vi "2_WF_Anomaly_Detection(Threshold_Evaluation).vi"() -> ()   [LabVIEW 2020]
uses:
  Controls/Optimal_Threshold_Range'.ctl
  <vilib>/Ngene/DeepLTK/Toolkit/NN_Network/subVIs/NN_Predict/NN_Predict(In1D_Out1D).vi
  <vilib>/Ngene/DeepLTK/Toolkit/NN_Data/subVIs/Get_Data_Vals/NN_Data_Get_ValByRef(2D_SGL).vi
  <vilib>/Ngene/DeepLTK/Toolkit/Deep_Learning_Toolkit_by_Ngene.lvlib
  <vilib>/Analysis/NI_AALPro.lvlib
panel:
  in  "Validation (Abnormal Samples) dataset path":path=path "D:/working/Anomaly Detection/Validation/Abnormal"
  in  "Validation (Normal Samples) dataset path":path=path "D:/working/Anomaly Detection/Validation/Normal"
  out "Integrals of Normalized Anomaly Score Distributions":cluster{"Axis":dbl[], "Integral X":dbl[]}[](graph)
  out "Anomaly Score Distribution":T1(graph)=[{"X Values"=array[700 elements], "Histogram: h(x)"=[0, 0, 0, 0, 0, 0, 0, 0, 0, 0, 0, 0, 0, 0, 0, 0, 0, 0, 0, 0, 0, 0, 0, 0, 0, 0, 0, 0, 0, 0, 0, 0, 0, 0, 0, 0, 1, 2, 5, 5, 8, 9, 5, 13, 9, 12, 13, 17, 13, 20, 12, 18, 18, 17, 20, 14, 17, 15, 19, 8, 9, 11, 14, 16, 9, 10, 16, 7, 6, 10, 10, 6, 9, 4, 4, 8, 3, 1, 5, 3, 2, 3, 5, 5, 3, 2, 3, 2, 2, 1, 4, 3, 0, 2, 0, 1, 1, 2, 3, 0, 1, 0, 0, 0, 0, 0, 0, 0, 0, 1, 0, 1, 1, 0, 0, 0, 0, 0, 0, 0, 1, 0, 0, 0, 0, 0, 0, 0, 0, 0, 0, 0, 0, 0, 0, 0, 0, 0, 0, 0, 0, 0, 0, 0, 0, 0, 0, 0, 0, 0, 0, 0, 0, 0, 0, 0, 0, 0, 0, 0, 0, 0, 0, 0, 0, 0, 0, 0, 0, 0, 0, 0, 0, 0, 0, 0, 0, 0, 0, 0, 0, 0, 0, 0, 0, 0, 0, 0, 0, 0, 0, 0, 0, 0, 0, 0, 0, 0, 0, 0, 0, 0, 0, 0, 0, 0, 0, 0, 0, 0, 0, 0, 0, 0, 0, 0, 0, 0, 0, 0, 0, 0, 0, 0, 0, 0, 0, 0, 0, 0, 0, 0, 0, 0, 0, 0, 0, 0, 0, 0, 0, 0, 0, 0, 0, 0, 0, 0, 0, 0, 0, 0, 0, 0, 0, 0, 0, 0, 0, 0, 0, 0, 0, 0, 0, 0, 0, 0, 0, 0, 0, 0, 0, 0, 0, 0, 0, 0, 0, 0, 0, 0, 0, 0, 0, 0, 0, 0, 0, 0, 0, 0, 0, 0, 0, 0, 0, 0, 0, 0, 0, 0, 0, 0, 0, 0, 0, 0, 0, 0, 0, 0, 0, 0, 0, 0, 0, 0, 0, 0, 0, 0, 0, 0, 0, 0, 0, 0, 0, 0, 0, 0, 0, 0, 0, 0, 0, 0, 0, 0, 0, 0, 0, 0, 0, 0, 0, 0, 0, 0, 0, 0, 0, 0, 0, 0, 0, 0, 0, 0, 0, 0, 0, 0, 0, 0, 0, 0, 0, 0, 0, 0, 0, 0, 0, 0, 0, 0, 0, 0, 0, 0, 0, 0, 0, 0, 0, 0, 0, 0, 0, 0, 0, 0, 0, 0, 0, 0, 0, 0, 0, 0, 0, 0, 0, 0, 0, 0, 0, 0, 0, 0, 0, 0, 0, 0, 0, 0, 0, 0, 0, 0, 0, 0, 0, 0, 0, 0, 0, 0, 0, 0, 0, 0, 0, 0, 0, 0, 0, 0, 0, 0, 0, 0, 0, 0, 0, 0, 0, 0, 0, 0, 0, 0, 0, 0, 0, 0, 0, 0, 0, 0, 0, 0, 0, 0, 0, 0, 0, 0, 0, 0, 0, 0, 0, 0, 0, 0, 0, 0, 0, 0, 0, 0, 0, 0, 0, 0, 0, 0, 0, 0, 0, 0, 0, 0, 0, 0, 0, 0, 0, 0, 0, 0, 0, 0, 0, 0, 0, 0, 0, 0, 0, 0, 0, 0, 0, 0, 0, 0, 0, 0, 0, 0, 0, 0, 0, 0, 0, 0, 0, 0, 0, 0, 0, 0, 0, 0, 0, 0, 0, 0, 0, 0, 0, 0, 0, 0, 0, 0, 0, 0, 0, 0, 0, 0, 0, 0, 0, 0, 0, 0, 0, 0, 0, 0, 0, 0, 0, 0, 0, 0, 0, 0, 0, 0, 0, 0, 0, 0, 0, 0, 0, 0, 0, 0, 0, 0, 0, 0, 0, 0, 0, 0, 0, 0, 0, 0, 0, 0, 0, 0, 0, 0, 0, 0, 0, 0, 0, 0, 0, 0, 0, 0, 0, 0, 0, 0, 0, 0, 0, 0, 0, 0, 0, 0, 0, 0, 0, 0, 0, 0, 0, 0, 0, 0, 0, 0, 0, 0, 0, 0, 0, 0, 0, 0, 0, 0, 0, 0, 0, 0, 0, 0, 0, 0, 0, 0, 0, 0, 0, 0, 0, 0, 0, 0, 0, 0, 0, 0, 0, 0, 0, 0, 0, 0, 0, 0, 0, 0, 0, 0, 0, 0, 0, 0, 0, 0, 0, 0, 0, 0, 0, 0, 0, 0, 0, 0, 0, 0]}, {"X Values"=array[700 elements], "Histogram: h(x)"=[0, 0, 0, 0, 0, 0, 0, 0, 0, 0, 0, 0, 0, 0, 0, 0, 0, 0, 0, 0, 0, 0, 0, 0, 0, 0, 0, 0, 0, 0, 0, 0, 0, 0, 0, 0, 0, 0, 0, 0, 0, 0, 0, 0, 0, 0, 0, 0, 0, 0, 0, 0, 0, 0, 0, 0, 0, 0, 0, 0, 0, 0, 0, 0, 0, 0, 0, 0, 0, 0, 0, 0, 0, 0, 0, 0, 0, 0, 0, 0, 0, 0, 0, 0, 0, 0, 0, 0, 0, 0, 0, 0, 0, 0, 0, 0, 0, 0, 0, 0, 0, 0, 0, 0, 0, 0, 0, 0, 0, 0, 0, 0, 0, 0, 0, 0, 0, 0, 0, 0, 0, 0, 0, 0, 0, 0, 0, 0, 0, 0, 0, 0, 0, 0, 0, 0, 0, 0, 0, 0, 0, 0, 0, 0, 0, 0, 0, 0, 0, 0, 0, 0, 0, 0, 0, 0, 0, 0, 0, 0, 0, 0, 0, 0, 0, 0, 0, 0, 0, 0, 0, 0, 1, 1, 0, 0, 0, 1, 0, 0, 1, 2, 2, 0, 0, 2, 1, 1, 2, 0, 0, 1, 2, 1, 2, 2, 1, 0, 1, 1, 2, 3, 0, 1, 2, 2, 2, 0, 2, 2, 1, 1, 2, 1, 2, 3, 0, 2, 3, 3, 5, 2, 2, 2, 1, 1, 0, 1, 7, 2, 0, 2, 1, 5, 1, 2, 2, 3, 0, 4, 0, 6, 2, 1, 3, 0, 2, 1, 0, 1, 6, 2, 2, 2, 1, 4, 2, 1, 4, 1, 4, 1, 0, 3, 1, 1, 2, 1, 1, 1, 1, 3, 2, 2, 2, 0, 1, 1, 3, 1, 1, 0, 2, 0, 2, 2, 1, 0, 1, 0, 3, 1, 0, 2, 1, 0, 0, 0, 0, 1, 0, 1, 1, 0, 1, 1, 1, 4, 1, 1, 0, 0, 1, 0, 2, 3, 2, 0, 0, 0, 1, 1, 1, 2, 2, 2, 1, 1, 0, 0, 0, 0, 1, 0, 2, 0, 0, 1, 1, 1, 1, 0, 1, 0, 1, 1, 1, 2, 1, 0, 1, 0, 1, 0, 1, 0, 1, 3, 3, 0, 1, 0, 1, 1, 1, 0, 0, 1, 0, 1, 0, 0, 2, 2, 2, 1, 0, 2, 0, 0, 1, 0, 0, 1, 3, 1, 2, 4, 1, 2, 2, 3, 3, 3, 3, 1, 1, 0, 2, 3, 1, 1, 1, 4, 5, 1, 4, 3, 0, 1, 1, 2, 1, 1, 1, 1, 0, 0, 0, 1, 1, 1, 0, 1, 0, 1, 3, 3, 0, 1, 0, 0, 0, 2, 2, 0, 3, 7, 3, 2, 1, 0, 0, 2, 2, 5, 0, 3, 0, 1, 1, 1, 2, 1, 2, 4, 0, 0, 0, 0, 0, 0, 2, 0, 2, 0, 1, 1, 0, 3, 0, 0, 0, 0, 0, 2, 1, 0, 0, 1, 1, 0, 0, 0, 0, 0, 0, 2, 0, 0, 0, 1, 0, 1, 0, 1, 0, 0, 0, 0, 0, 0, 0, 0, 0, 0, 0, 0, 0, 0, 0, 0, 0, 0, 0, 0, 0, 0, 0, 0, 0, 0, 0, 0, 1, 0, 0, 0, 0, 0, 0, 0, 0, 0, 0, 0, 0, 0, 0, 0, 0, 0, 0, 0, 0, 0, 0, 0, 0, 1, 0, 0, 0, 0, 0, 1, 1, 0, 0, 0, 0, 3, 1, 1, 1, 0, 1, 1, 0, 0, 1, 1, 2, 4, 0, 0, 0, 0, 1, 0, 1, 1, 1, 0, 0, 3, 0, 0, 1, 2, 1, 0, 1, 3, 3, 0, 1, 1, 2, 0, 2, 0, 2, 1, 1, 1, 3, 4, 0, 1, 2, 2, 2, 5, 1, 1, 2, 2, 0, 2, 2, 2, 1, 3, 0, 3, 2, 0, 0, 0, 0, 0, 0, 0, 1, 2, 3, 0, 2, 1, 0, 1, 0, 0, 1, 0, 0, 0, 0, 0, 0, 0, 0, 0, 0, 0, 0, 0, 1, 0, 0, 0, 0, 0, 0, 0, 0, 0, 0, 0, 0, 0, 0, 0, 0, 0, 0, 0, 0, 0, 0, 0, 0, 0, 0, 0, 0, 0, 0, 0, 0, 0, 0, 0, 0, 0, 0, 0, 0, 0]}]
  out "Optimal Threshold Range":T2={"Start"=0.17357142857142857, "Stop"=0.245}
  in  "Weights File Path":path=path "D:/Ngene/GitHub/deepltk_examples/2_Waveform_Processing/24_Waveform_Anomaly_Detection/working/Anomaly_Detection/Anomaly_Detection_weights_24_01_10__18_49_12.bin"
  in  "CFG file path":path=path "D:/Ngene/GitHub/deepltk_examples/2_Waveform_Processing/24_Waveform_Anomaly_Detection/working/Anomaly_Detection/Anomaly_Detection_net_cfg_24_01_10__18_49_12.cfg"
  # "Overview: This VI is designed to calculate the optimal anomaly threshold on the generated synthetic dataset.\nRequirements: Deep Learning Toolkit for LabVIEW - https://www.ngene.co/deep-learning-toolkit-for-labview\nInstructions:\n1. Provide \"Network Configuration File Path\" and \"Weight File Path\" generated from \"1_WF_Anomaly_Detection(Training).vi\".\n2. Provide Validation (Normal Samples) and Validation (Abnormal Samples) dataset paths.\n3. Run the VI.\n4.Observe the Range of optimal threshold values.\n5. Choose a value from the range of optimal threshold calculated after the VI stops, and use it as a anomaly detetcion threshold in \"3_Waveform_Anomaly_Detection(Inference).vi\" \n6. Open \"3_WF_Anomaly_Detection(Accuracy_Evaluation).vi\"  to deploy the trained network for inference."
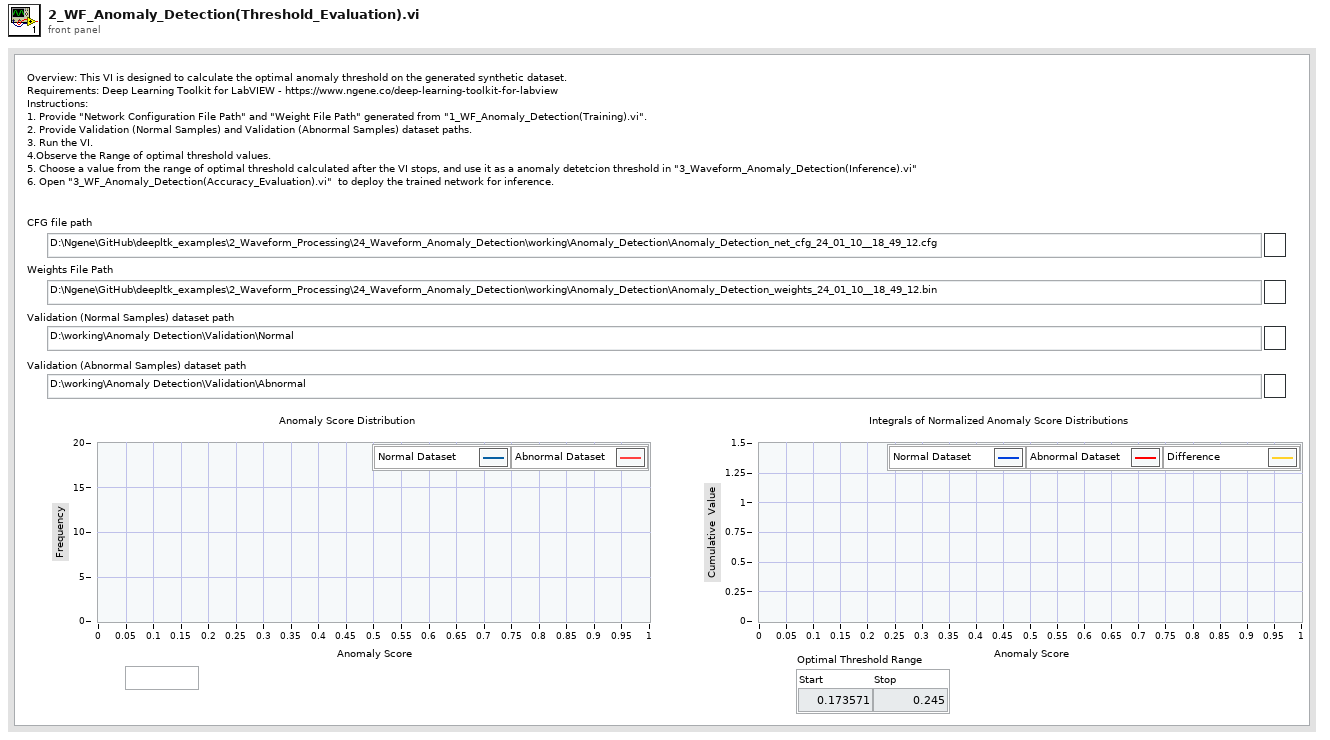
[diagram p1: front panel]
types:
  T1 = cluster{"X Values":dbl[], "Histogram: h(x)":i32[]}[]
  T2 = typedef "Optimal_Threshold_Range'.ctl" = cluster{"Start":dbl, "Stop":dbl}
  T3 = typedef "Deep_Learning_Toolkit_by_Ngene.lvlib/NN_Config_Params.ctl" = cluster{"Name":string, "mBatch":i32, "NN_Train_Params":T4, "LR_Decay_Policy":T7, "Labels":string[], "Loss":T9}
  T4 = typedef "Deep_Learning_Toolkit_by_Ngene.lvlib/NN_Train_Params.ctl" = cluster{"Optimizer":T5, "Beta_1":sgl, "Beta_2":sgl, "Weight Decay(L1)":sgl, "Weight Decay(L2)":sgl, "Data_Sampling":T6}
  T5 = typedef "Deep_Learning_Toolkit_by_Ngene.lvlib/NN_Train_Optimizer.ctl" = enum16{"SGD", "Adam", "Adagrad", "Adadelta", "RMSProp", "Nesterov"}
  T6 = typedef "Deep_Learning_Toolkit_by_Ngene.lvlib/NN_Train_Data_Sampling.ctl" = enum16{"Random", "Sequential"}
  T7 = typedef "Deep_Learning_Toolkit_by_Ngene.lvlib/NN_LR_Policy_Cfg.ctl" = cluster{"Policy_Type":T8, "LR0":dbl, "k":sgl, "WarmUp_Policy":enum16{"Step", "Ramp"}, "WarmUp_Iter":i32, "WarmUp_Ratio":sgl}
  T8 = typedef "Deep_Learning_Toolkit_by_Ngene.lvlib/NN_LR_Policy_Type.ctl" = enum16{"Manual", "Step", "Exp", "1/t"}
  T9 = typedef "Deep_Learning_Toolkit_by_Ngene.lvlib/NN_Loss_Config_Params.ctl" = cluster{"Loss_Type":T10, "Loss_Conf_Params":variant}
  T10 = typedef "Deep_Learning_Toolkit_by_Ngene.lvlib/NN_Loss_Type.ctl" = enum16{"None", "MSE", "CrossEntropy", "YOLO_v2"}
  T11 = typedef "Deep_Learning_Toolkit_by_Ngene.lvlib/NN_Layer_Config_Params.ctl" = cluster{"Layer_Type":T12, "Layer_Conf_Params":variant}
  T12 = typedef "Deep_Learning_Toolkit_by_Ngene.lvlib/NN_Layer_Type.ctl" = enum16{"Input1D", "Input3D", "Conv2D", "Conv2D_Adv", "MaxPool", "AvgPool", "UpSample", "DropOut3D", "ShortCut", "Concat", "SoftMax3D", "FC", "DropOut", "Softmax", "Flatten", "YOLO_v2", "Unsupported"}
  T13 = typedef "Deep_Learning_Toolkit_by_Ngene.lvlib/NN.ctl" = cluster{"Name":string, "No of Layers":i32, "mBatch":i32, "Layers":T14[], "Dimty":T15, "Dims_In":T16, "Dims_Out":T16, "Working_Dir":path, "Train?":bool, "Train_Params":T4, "LR_Update_Policy":T7, "Session Data":T17, "Ground_truth":T18, "NNg_hdls":T20, "NN_Device":T21, "GPU Id":i32, "Labels":string[], "Receptive Field":T22[], "Loss_Type":T10, "Loss_Cfg_Prms":variant}
  T14 = typedef "Deep_Learning_Toolkit_by_Ngene.lvlib/NN_Layer_ref.ctl" = refnum<data-value>
  T15 = typedef "Deep_Learning_Toolkit_by_Ngene.lvlib/NN_In_Out_Dim-ty.ctl" = enum8{"In1D_Out1D", "In3D_Out1D", "In3D_Out3D", "In3D_OutBBox"}
  T16 = typedef "Deep_Learning_Toolkit_by_Ngene.lvlib/NN_Dims(C,H,W).ctl" = cluster{"C":i32, "H":i32, "W":i32}
  T17 = typedef "Deep_Learning_Toolkit_by_Ngene.lvlib/NN_Train_Session_Data.ctl" = cluster{"Epochs":sgl, "Tot_Iter":i32, "LR":sgl, "LR_iter":i32}
  T18 = typedef "Deep_Learning_Toolkit_by_Ngene.lvlib/NN_Ground_truth.ctl" = cluster{"Y":variant, "Y_idx":T19}
  T19 = typedef "Deep_Learning_Toolkit_by_Ngene.lvlib/NN_Data_ref(1D_I32).ctl" = refnum<data-value>
  T20 = typedef "Deep_Learning_Toolkit_by_Ngene.lvlib/nng_cuda_handles.ctl" = cluster{"cudnn":u64, "cublas":u64, "stream":u64, "curand":u64}
  T21 = typedef "Deep_Learning_Toolkit_by_Ngene.lvlib/NN_Device.ctl" = enum16{"CPU", "GPU"}
  T22 = typedef "Deep_Learning_Toolkit_by_Ngene.lvlib/NN_Dims(V,H).ctl" = cluster{"V":i32, "H":i32}
  T23 = typedef "Deep_Learning_Toolkit_by_Ngene.lvlib/NN_DataSet(In1D_Out1D).ctl" = cluster{"Inputs Ref.":T24, "Outputs Ref.":T24, "Dims_In":i32, "Dataset_Size":i32, "Outputs_idx Ref.":T19, "Dims_Out":i32, "Labels":string[], "File Paths":path[]}
  T24 = typedef "Deep_Learning_Toolkit_by_Ngene.lvlib/NN_Data_ref(2D_SGL).ctl" = refnum<data-value>
  T25 = cluster{"X Values":dbl[], "Histogram: h(x)":i32[]}
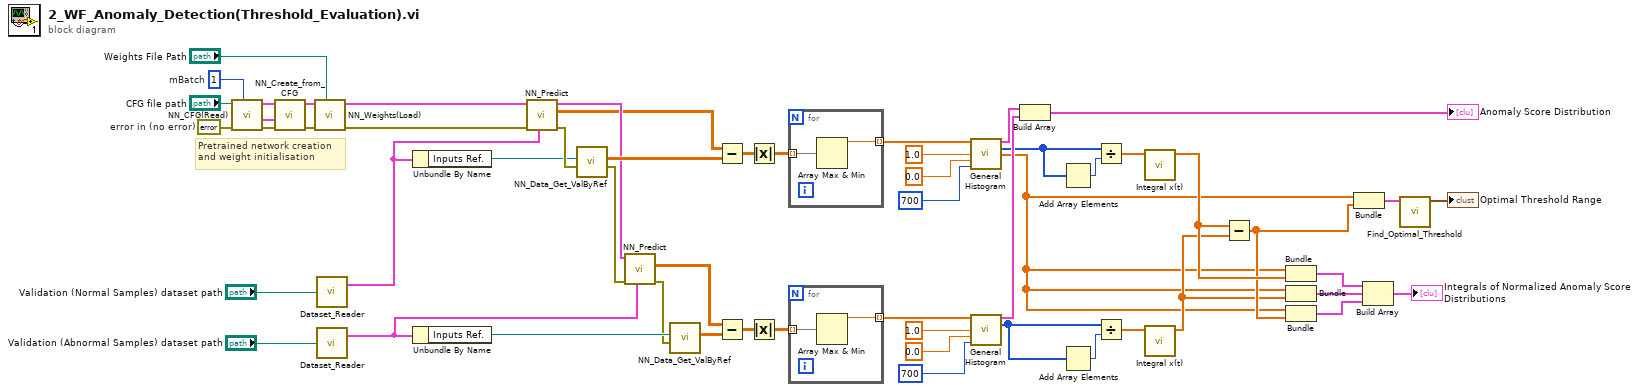
[diagram p0: block diagram]
diagram:
  w50 = 1  # mBatch
  w55 = errorcluster {"status"=FALSE, "code"=0, "source"=""}  # error in (no error)
  # "Pretrained network creation\nand weight initialisation"
  n1 = call <vilib>:"NN_CFG(Read).vi"("mBatch"=w50, "error in (no error)"=w55, "CFG file path"="CFG file path") -> ("error out"=w53:errorcluster, "Net_Cfg"=w54:T3, "Layer_Cfg"=w52:T11[])  [unwired: 6 in]
  n2 = call <vilib>:"NN_Create_from_CFG.vi"("error in (no error)"=w53, "Net_Cfg"=w54, "Layer_Cfg"=w52) -> ("error out"=w56:errorcluster, "NN out"=w51:T13)  [unwired: 7 in]
  n3 = call <vilib>:"NN_Weights(Load).vi"("Weight File Path"="Weights File Path", "error in (no error)"=w56, "NN in"=w51) -> ("error out"=w17:errorcluster, "NN out"=w18:T13)  [unwired: 7 in]
  n4 = call "Dataset_Reader.vi"("Train dataset path"="Validation (Normal Samples) dataset path") -> ("Dataset"=w6:T23)  [unwired: 2 in, 1 out]
  n5 = call "Dataset_Reader.vi"("Train dataset path"="Validation (Abnormal Samples) dataset path") -> ("Dataset"=w7:T23)  [unwired: 2 in, 1 out]
  n6 = Unbundle By Name(w6) -> ("Inputs Ref."=w5:T24)
  n7 = Unbundle By Name(w7) -> ("Inputs Ref."=w41:T24)
  n8 = call-poly <vilib>:"NN_Predict.vi"("Dataset"=w6, "error in (no error)"=w17, "NN in"=w18) -> ("error out"=w47:errorcluster, "Predictions"=w37:sgl[][], "NN out"=w43:T13)  [unwired: 6 in]
  n9 = call-poly <vilib>:"NN_Data_Get_ValByRef.vi"("error in (no error)"=w47, "DVR(2D_SGL)"=w5) -> ("error out"=w44:errorcluster, "Value(2D_SGL)"=w46:sgl[][])  [unwired: 6 in]
  n10 = call-poly <vilib>:"NN_Predict.vi"("Dataset"=w7, "error in (no error)"=w44, "NN in"=w43) -> ("error out"=w40:errorcluster, "Predictions"=w38:sgl[][])  [unwired: 6 in, 1 out]
  n11 = call-poly <vilib>:"NN_Data_Get_ValByRef.vi"("error in (no error)"=w40, "DVR(2D_SGL)"=w41) -> ("Value(2D_SGL)"=w39:sgl[][])  [unwired: 6 in, 1 out]
  n12 = Subtract(x=w37, y=w46) -> (x-y=w45:sgl[][])
  n13 = Subtract(x=w38, y=w39) -> (x-y=w42:sgl[][])
  n14 = Absolute Value(x=w45) -> (abs(x)=w36:sgl[][])
  n15 = Absolute Value(x=w42) -> (abs(x)=w35:sgl[][])
  n16 = for {
    tunnel: w36 -> [w58] mode=indexing
    tunnel: [w57] -> w8 mode=indexing
    n17 = Array Max & Min(array=w58) -> (max value=w57:sgl)  [unwired: 3 out]
  }
  n18 = for {
    tunnel: w35 -> [w60] mode=indexing
    tunnel: [w59] -> w9 mode=indexing
    n19 = Array Max & Min(array=w60) -> (max value=w59:sgl)  [unwired: 3 out]
  }
  n20 = call <vilib>:"General Histogram.vi"("X"=w8, "max"=1.0, "min"=0.0, "# bins"=700) -> ("Histogram Graph"=w23:T25, "Histogram"=w21:i32[], "Axis"=w10:dbl[])  [unwired: 7 in, 2 out]
  n21 = call <vilib>:"General Histogram.vi"("X"=w9, "max"=1.0, "min"=0.0, "# bins"=700) -> ("Histogram Graph"=w22:T25, "Histogram"=w26:i32[])  [unwired: 7 in, 3 out]
  n22 = Build Array(w23, w22) -> (→"Anomaly Score Distribution":T1)
  n23 = Add Array Elements(numeric array=w21) -> (sum=w24:i32)
  n24 = Add Array Elements(numeric array=w26) -> (sum=w25:i32)
  n25 = Divide(x=w21, y=w24) -> (x/y=w27:dbl[])
  n26 = Divide(x=w26, y=w25) -> (x/y=w28:dbl[])
  n27 = call <vilib>:"Integral x(t).vi"("X"=w27) -> ("Integral X"=w15:dbl[])  [unwired: 9 in, 1 out]
  n28 = call <vilib>:"Integral x(t).vi"("X"=w28) -> ("Integral X"=w13:dbl[])  [unwired: 9 in, 1 out]
  n29 = Subtract(x=w15, y=w13) -> (x-y=w14:dbl[])
  n30 = Bundle("Axis"=w10, "Integral X"=w15) -> (w1:cluster{"Axis":dbl[], "Integral X":dbl[]})  [unwired: 1 in]
  n31 = Bundle("Axis"=w10, "Integral X"=w13) -> (w2:cluster{"Axis":dbl[], "Integral X":dbl[]})  [unwired: 1 in]
  n32 = Bundle("Axis"=w10, w14) -> (w12:cluster{"Axis":dbl[], dbl[]})  [unwired: 1 in]
  n33 = Bundle("Axis"=w10, w14) -> (w20:cluster{"Axis":dbl[], dbl[]})  [unwired: 1 in]
  n34 = Build Array(w1, w2, w12) -> (→"Integrals of Normalized Anomaly Score Distributions":cluster{"Axis":dbl[], "Integral X":dbl[]}[])
  n35 = call "Find_Optimal_Threshold.vi"("0000000 4"=w20) -> ("Optimal Threshold"=→"Optimal Threshold Range":T2)  [unwired: 10 in]
